vi "rqp_Start Exiting.vi"(7 "Caller in":refnum<class "Worker.lvclass">, 8 "error in":errorcluster, 11 "sequenceManagerWorker in":refnum<class "sequenceManagerWorker.lvclass">) -> (0 "error out":errorcluster, 3 "dup sequenceManagerWorker out":refnum<class "sequenceManagerWorker.lvclass">, 5 "dup Caller out":refnum<class "Worker.lvclass">)   [LabVIEW 2023, in "sequenceManagerWorker.lvclass"]
doc: "This VI will indirectly send a message to the <Start Exiting> MHL case of the Worker that own this VI.\n---\nThe shutdown sequence of the Worker that owns this VI will be initiated."
uses:
  sequenceManagerWorker.lvclass
  <vilib>/addons/_Workers/Library/Classes/Worker/Worker.lvclass
  <vilib>/addons/_Workers/Library/Classes/Message Queue/Message Queue.lvclass
  sequenceManagerWorker.lvclass/sequenceManagerWorker.ctl
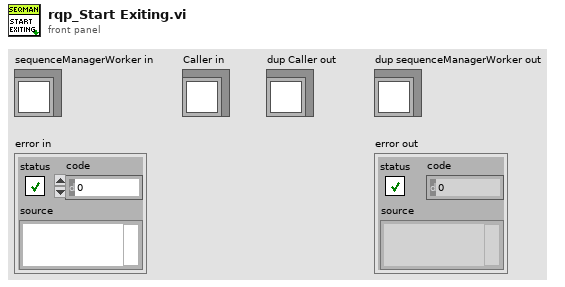
[diagram p1: front panel]
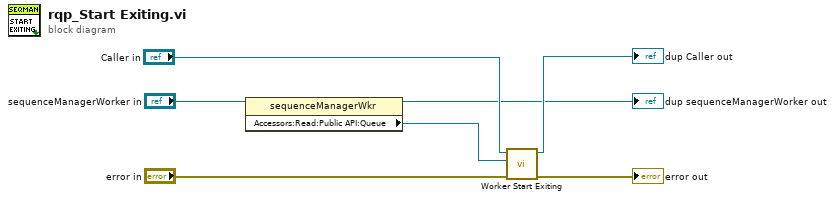
[diagram p0: block diagram]
diagram:
  n1 = property class="sequenceManagerWkr"(reference="sequenceManagerWorker in") -> (reference out=→"dup sequenceManagerWorker out":refnum<class "sequenceManagerWorker.lvclass">, "Accessors:Read:Public API:Queue"=w1:refnum<class "Message Queue.lvclass">)  [unwired: 1 in, 1 out]
  n2 = call-dynamic "Worker Start Exiting.vi"("error_in"="error in", "Message Queue"=w1, "Worker"="Caller in") -> ("error out"=→"error out":errorcluster, "dup Worker out"=→"dup Caller out":refnum<class "Worker.lvclass">)  [unwired: 7 in]
